vi "DiscArchiver.get archive status.vi"(0 "i ref in":refnum<vi>, 5 "error in (no error)":errorcluster) -> (14 "i ref out":refnum<vi>, 15 "actual file":string, 16 "# of items":i32, 18 "eventBuilder":string, 19 "error out":errorcluster)   [LabVIEW 2014, in "DiscArchiver.lvlib"]
doc: "gets the status of the DiscArchiver object."
uses:
  DiscArchiver.lvlib
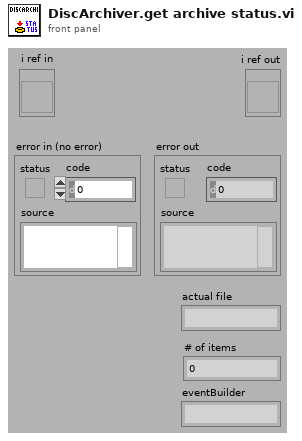
[diagram p1: front panel]
types:
  T1 = typedef "DiscArchiver.lvlib/DiscArchiver.i attribute.ctl" = cluster{"file prefix":string, "actual file":string, "nOfEvents":i32, "file":refnum<file>, "eventBuilder":string, "disc size alarm":bool, "dataDescription":string, "dataDescriptionURL":string, "eventDataURL":string, "headerID":dbl, "completeData":bool, "nOfEventsID":i32, "dataFileID":i32}
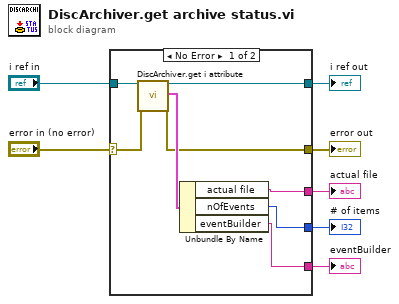
[diagram p0: block diagram]
diagram:
  n1 = case shown="No Error" "error in (no error)" {
    selector: "error in (no error)" -> [w8 w16]
    tunnel: "i ref in" -> [w15 w17]
    tunnel: [w13 w17] -> w6
    tunnel: [w12 w16] -> w5
    tunnel: [w11 _] -> w4
    tunnel: [w10 _] -> w3
    tunnel: [w9 _] -> w2
    frame No Error {
      n2 = call "DiscArchiver.get i attribute.vi"("i ref in"=w15, "error in (no error)"=w8) -> ("i ref out"=w13:refnum<vi>, "i attribute"=w14:T1, "error out"=w12:errorcluster)  [unwired: 15 in]
      n3 = Unbundle By Name(w14) -> ("actual file"=w11:string, "nOfEvents"=w10:i32, "eventBuilder"=w9:string)
    }
    frame Error {
    }
  }
  "error out" <- w5
  "i ref out" <- w6
  "actual file" <- w4
  "# of items" <- w3
  "eventBuilder" <- w2
